vi "msg.available_lua.vi"(5 "LuaVIEW reference":T1) -> (15 "error out":errorcluster)   [LabVIEW 2012]
doc: "Checks wether there are one or more messages available in the task's message queue.\nResults:\nbool:available\nErrors:\nFunction must be called from a task context but was not."
uses:
  typedefs/t_LuaVIEW Reference.ctl
  typedefs/t_LuaVIEW Task State Methods.ctl
  subvis/private/LuaVIEW Push (boolean).vi
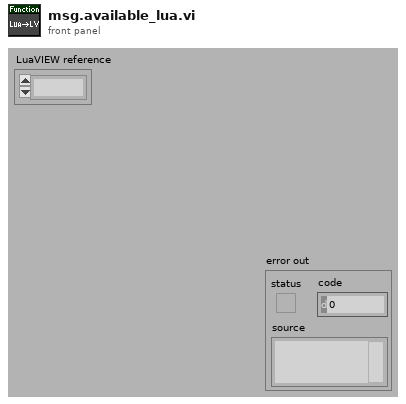
[diagram p1: front panel]
types:
  T1 = typedef "t_LuaVIEW Reference.ctl" = refnum<k1>
  T2 = typedef "t_LuaVIEW Task State Methods.ctl" = enum16{"cleanup", "set initial", "set mode", "set active mode", "set error", "get task info", "get script info", "set signal", "clear signal", "test handled", "test delegated", "test signal", "handle signal", "delegate signal", "allow signal", "disallow signal", "disallow all", "signals?", "delegated signals?", "protection++", "protection--", "protection=0", "message", "next message", "pop message", "message available?", "force stop", "set swap preps", "apply swap preps"}
  T3 = typedef "t_LuaVIEW Task State Pane.ctl" = refnum<vi>
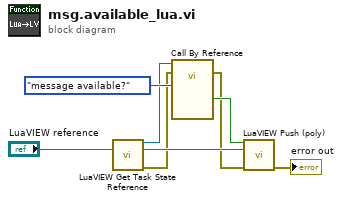
[diagram p0: block diagram]
diagram:
  n1 = call "LuaVIEW Get Task State Reference.vi"("LuaVIEW reference in"="LuaVIEW reference") -> ("task state reference"=w6:T3, "LuaVIEW reference out"=w7:T1, "error out"=w4:errorcluster)  [unwired: 12 in]
  n2 = call-by-ref "?"(reference=w6, error in=w4, "method"=t_LuaVIEW_Task_State_Methods."message available?") -> (error out=w1:errorcluster, "set/available/pending"=w3:bool)  [unwired: 10 in, 5 out]
  n3 = call-poly "LuaVIEW Push (poly).vi"("boolean"=w3, "LuaVIEW reference in"=w7, "error in (no error)"=w1) -> ("error out"=→"error out":errorcluster)  [unwired: 11 in, 1 out]
